vi "Add JSONable object to JSON Tree.vi"(8 "error in (no error)":errorcluster, 9 "Name":string, 10 "JSONable in":refnum<class "JSONable.lvclass">, 11 "JSON Tree in (JSON Object)":variant) -> (0 "error out":errorcluster, 3 "JSON Tree out (JSON Object)":variant)   [LabVIEW 2015]
uses:
  JSONable.lvclass
  <vilib>/NI/i3 JSON/JSON Generation/Add Object Parameter Files/Add Object Parameter - Known Type.vi
  <vilib>/NI/i3 JSON/i3-json.lvlib
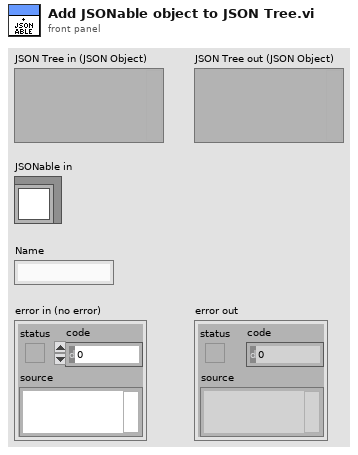
[diagram p1: front panel]
types:
  T1 = typedef "i3-json.lvlib/JSON Type.ctl" = enum8{"JSON Compatible", "JSON Array", "JSON Object", "JSON Null", "Double", "String", "Boolean", "Unknown"}
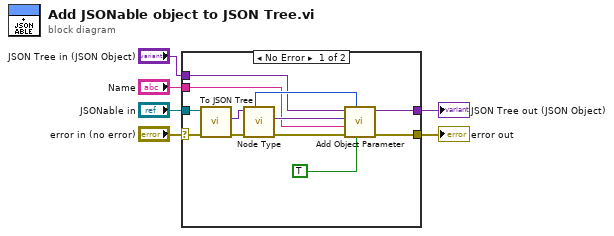
[diagram p0: block diagram]
diagram:
  n1 = case shown="No Error" "error in (no error)" {
    selector: "error in (no error)" -> [w9 w20]
    tunnel: [w8 w20] -> w5
    tunnel: "JSONable in" -> [w13 _]
    tunnel: "JSON Tree in (JSON Object)" -> [w12 w19]
    tunnel: [w11 w19] -> w2
    tunnel: "Name" -> [w10 _]
    frame No Error {
      n2 = call-dynamic "To JSON Tree.vi"("error in (no error)"=w9, "JSONable in"=w13) -> ("error out"=w15:errorcluster, "JSON Tree Out"=w18:variant)  [unwired: 7 in, 1 out]
      n3 = call <vilib>:"Node Type.vi"("error in (no error)"=w15, "JSON Tree In"=w18) -> ("error out"=w14:errorcluster, "Value"=w16:variant, "JSON Type"=w17:T1)  [unwired: 5 in, 2 out]
      n4 = call-poly <vilib>:"Add Object Parameter.vi"("Add Parameter as JSON Tree?"=TRUE, "JSON Type"=w17, "error in (no error)"=w14, "Name"=w10, "Value"=w16, "JSON Tree in (JSON Object)"=w12) -> ("error out"=w8:errorcluster, "JSON Tree out (JSON Object)"=w11:variant)  [unwired: 4 in]
    }
    frame Error {
    }
  }
  "error out" <- w5
  "JSON Tree out (JSON Object)" <- w2
